vi "ClientUDP.vi"() -> ()   [LabVIEW 2020]
panel:
  out "koniec":bool
  out "Waveform Graph":dbl[](graph)
  out "seconds since 1Jan1904":timestamp
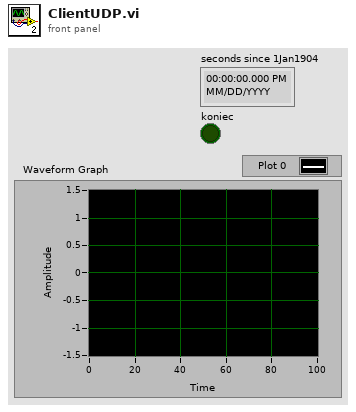
[diagram p1: front panel]
types:
  T1 = typedef "Wiasomoœæ_c.ctl" = cluster{"seconds since 1Jan1904":timestamp, "Y":dbl[], bool}
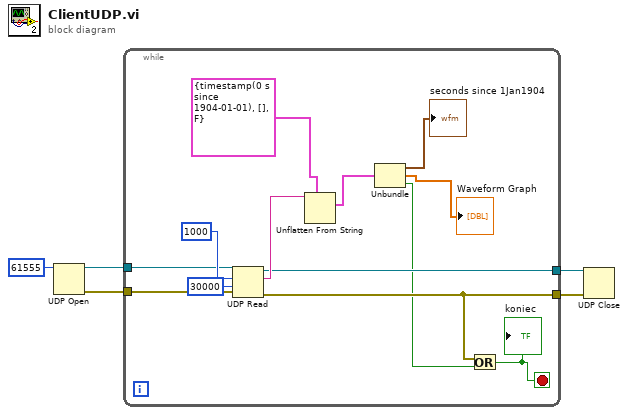
[diagram p0: block diagram]
diagram:
  n1 = UDP Open(11:u16 61555 ("port")) -> (port=w4:refnum<k16>, 0:w2:errorcluster)  [unwired: 4 in, 1 out]
  n2 = while {
    tunnel: w4 -> [w15]
    tunnel: [w14] -> w3
    tunnel: w2 -> [w13]
    tunnel: [w12] -> w1
    stop <- w11 stop-if-true
    n3 = UDP Read(connection ID=w15, max size (548)=1000, timeout ms (25000)=30000, 8:w13) -> (data out=w16:string, error out=w12:errorcluster, 3:w14:refnum<k16>)  [unwired: 2 out]
    n4 = Unflatten From String(type=T1 {"seconds since 1Jan1904"=timestamp(0 s since 1904-01-01), "Y"=[], FALSE} ("output cluster"), binary string=w16) -> (value=w10:T1)  [unwired: 3 in, 2 out]
    n5 = Unbundle(w10) -> ("seconds since 1Jan1904"=→"seconds since 1Jan1904":timestamp, "Y"=→"Waveform Graph":dbl[], w7:bool)
    n6 = Or(x=w12, y=w7) -> (x .or. y?=w11:bool)
    "koniec" <- w11
  }
  n7 = UDP Close(connection ID=w3, 8:w1) -> ()  [unwired: 2 out]
